vi "about read tMasterInformation ODBC.vi"(8 "error in (no error)":errorcluster, 11 "DF Index db (\"\")":path) -> (0 "error out":errorcluster, 2 "values":string[](array[string]), 3 "names":string[](array[string]))   [LabVIEW 2011]
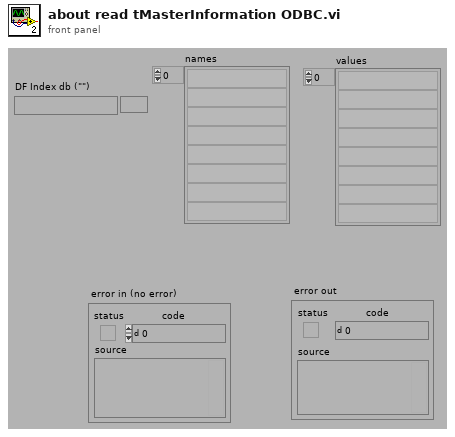
[diagram p1: front panel]
types:
  T1 = typedef "Connection Refnum.ctl" = cluster{"Environment Handle":i32, "Connection Handle":i32}
  T2 = typedef "Statement Refnum.ctl" = cluster{"Statement Handle":i32, "Parameter Number":u16}
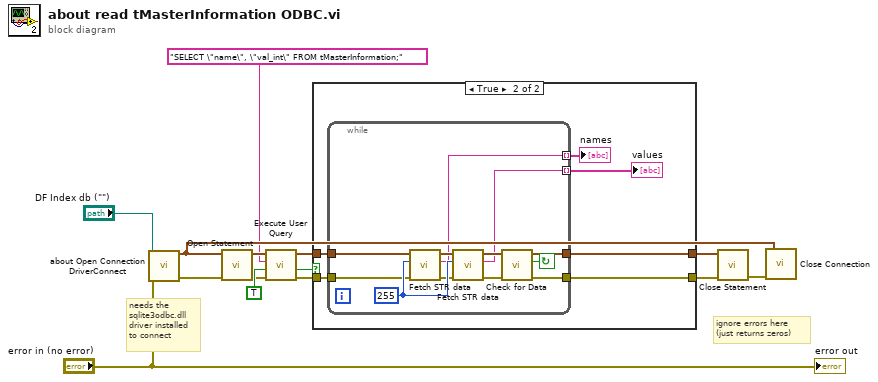
[diagram p0: block diagram]
diagram:
  # "ignore errors here\n(just returns zeros)"
  # "needs the\nsqlite3odbc.dll\ndriver installed\nto connect"
  n1 = call "about Open Connection DriverConnect.vi"("error in (no error)"="error in (no error)", "ODBC Database (\"\")"="DF Index db (\"\")") -> ("error out"=w3:errorcluster, "Connection Refnum"=w6:T1)  [unwired: 5 out]
  n2 = call "Open Statement.vi"("error in (no error)"=w3, "Connection Refnum"=w6) -> ("error out"=w9:errorcluster, "Statement Refnum"=w10:T2)  [unwired: 4 out]
  n3 = call "Execute User Query.vi"("error in (no error)"=w9, "Return Data? (f)"=TRUE, "User Query"="SELECT \"name\", \"val_int\" FROM tMasterInformation;" ("Query Name"), "Statement Refnum"=w10) -> ("error out"=w13:errorcluster, "Data Present?"=w14:bool, "Statement Refnum"=w12:T2)  [unwired: 1 out]
  n4 = case shown="True" w14 {
    tunnel: w13 -> [w15 w22]
    tunnel: w12 -> [w16 w21]
    tunnel: [w15 w20] -> w8
    tunnel: [w16 w19] -> w7
    frame False {
    }
    frame True {
      n5 = while {
        tunnel: w22 -> [w25]
        tunnel: w21 -> [w26]
        tunnel: [w33] -> w20
        tunnel: [w32] -> w19
        tunnel: [w24] -> w18 mode=indexing
        tunnel: [w23] -> w17 mode=indexing
        stop <- w34 continue-if-true
        w31 = 255 ("Buffer Size")
        n6 = call "Fetch STR data.vi"("error in (no error)"=w25, "Buffer Size"=w31, "Statement Refnum"=w26) -> ("error out"=w30:errorcluster, "Data"=w24:string, "Statement Refnum"=w29:T2)  [unwired: 2 out]
        n7 = call "Fetch STR data.vi"("error in (no error)"=w30, "Buffer Size"=w31, "Statement Refnum"=w29) -> ("error out"=w27:errorcluster, "Data"=w23:string, "Statement Refnum"=w28:T2)  [unwired: 2 out]
        n8 = call "Check for Data.vi"("error in (no error)"=w27, "Statement Refnum"=w28) -> ("error out"=w33:errorcluster, "Data Present?"=w34:bool, "Statement Refnum"=w32:T2)  [unwired: 3 out]
      }
      "names" <- w18
      "values" <- w17
    }
  }
  n9 = call "Close Statement.vi"("error in (no error)"=w8, "Statement Refnum"=w7) -> ("error out"=w5:errorcluster)  [unwired: 5 out]
  n10 = call "Close Connection.vi"("error in (no error)"=w5, "Connection Refnum"=w6) -> ()  [unwired: 6 out]
  "error out" <- "error in (no error)"
